vi "R.E.D.vi"(0 "A":T1, 1 "B":dbl[](array[numeric]), 2 "C":dbl[](array[numeric]), 3 "u(k)":dbl, 4 "Retardo":dbl) -> (5 "x(k)":dbl[](array[numeric]), 6 "Y(kt)":dbl format="%.2f")   [LabVIEW 2019]
doc: "R.E.D\nRespuesta en espacio de estados para sistemas discretos. \nCreadores.\nJuan Ricardo Cardona.\nDiego Alejandro Henao Jiménez.\nPolitécnico JIC.\nEste Sub-Vi parte de las dos ecuaciones que permiten visualizar el estado de un sistema discreto de acuerdo a una estimulación, las ecuaciones son: \n1) x(k+1)=Ax(k)+Bu(k) (Ecuacion de Entrada)\n2) y(k)=Cx(k)+Du(k) (Ecuacion de salida)\n Estan tienen como entradas:\n A: Matriz de dimensión N*N, llamada matriz del sistema. \nB: vector de entradas de dimensión (N*R).\nC: vector de salidas de dimensión (M*R).\nU(k): escalar que sirve como estimulación. \nTiene como salidas:\n X(k): Vector de estado de dimensión (N).\nY(k): Vector de salida de dimensión (N)."
uses:
  <vilib>/Analysis/Matrix/Datatypes/RealMatrix.ctl
  <vilib>/Analysis/baseanly.llb/Real Dot Product.vi
  <vilib>/Analysis/baseanly.llb/A x Vector.vi
  <menus>/Categories/IAControl Library/continuous linear.llb/Integrator (DBL Array).vi
  <vilib>/Analysis/NI_AALBase.lvlib
  <vilib>/Analysis/Matrix/NI_Matrix.lvlib
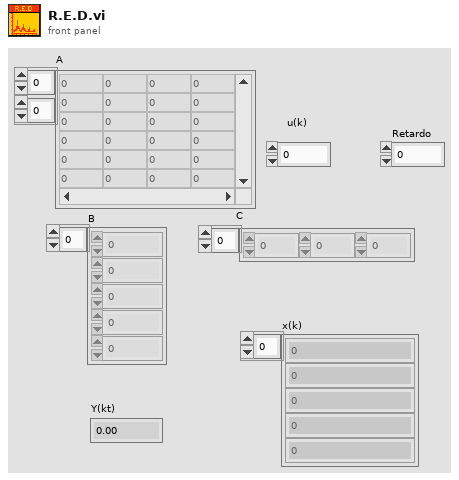
[diagram p1: front panel]
types:
  T1 = typedef "NI_Matrix.lvlib/RealMatrix.ctl" = dbl[][]
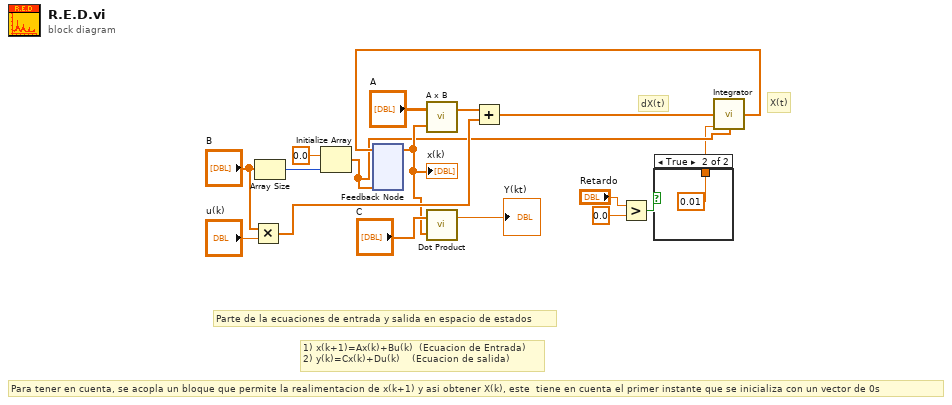
[diagram p0: block diagram]
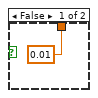
[diagram p2: hidden frame]
diagram:
  # "X(t)"
  # "dX(t)"
  # "Para tener en cuenta, se acopla un bloque que permite la realimentacion de x(k+1) y asi obtener X(k), este  tiene en cuenta el primer instante que se inicializa con un vector de 0s"
  # "1) x(k+1)=Ax(k)+Bu(k)  (Ecuacion de Entrada)\n2) y(k)=Cx(k)+Du(k)    (Ecuacion de salida)"
  # "Parte de la ecuaciones de entrada y salida en espacio de estados"
  n1 = Multiply(x="B", y="u(k)") -> (x*y=w15:dbl[])
  n2 = Array Size(array="B") -> (size(s)=w8:i32)
  n3 = Initialize Array(0.0 ("element"), w8) -> (w5:dbl[])
  n4 = feedback #1(w5) -> (w9:dbl[])
  "x(k)" <- w9
  n5 = call-poly <vilib>:"A x B.vi"("Vector"=w9, "A"="A") -> ("A x Vector"=w14:dbl[])  [unwired: 1 out]
  n6 = call-poly <vilib>:"Dot Product.vi"("Y Vector"=w9, "X Vector"="C") -> ("X * Y"=→"Y(kt)":dbl)  [unwired: 1 out]
  n7 = Add ("Add.vi")(x=w14, y=w15) -> (x+y=w7:dbl[])
  n8 = Greater?(x="Retardo", y=0.0) -> (0:w1:bool)
  n9 = case shown="True" w1 {
    tunnel: [0.01 ("y") 0.01 ("dt")] -> w4
    frame False {
    }
    frame True {
    }
  }
  n10 = call-poly <menus>:"Integrator.vi"("input points"=w7, "dt"=w4, "initial conditions"=w5) -> ("output points"=w6:dbl[])  [unwired: 12 in]
  n11 = feedback-in #1(w6) -> ()
